vi "Apply Voltage.vi"(8 "error in (no error)":errorcluster, 10 "Number of Points":i32, 11 "Tool Path in":refnum<class "Tool Path.lvclass">) -> (0 "error out":errorcluster, 2 "Voltage Values":dbl[](array[numeric]), 3 "Tool Path out":refnum<class "Tool Path.lvclass">)   [LabVIEW 2019, in "Tool Path.lvclass"]
uses:
  Tool Path.lvclass
  subVIs/typedefs/Schedule - enum.ctl
  Settings/ObjectSettings/ObjectSettings.lvclass/ObjectSettings.ctl
  subVIs/typedefs/Schedule Types/Schedule--Constant.ctl
  subVIs/typedefs/Schedule Types/Schedule--Ramp.ctl
  subVIs/typedefs/Schedule Types/Schedule--Function Generator.ctl
  subVIs/typedefs/Schedule Types/Schedule--Formula.ctl
  Settings/Path Settings/Path Settings.lvclass
  C:/Users/Albro/Documents/GitHub/AFM-Lithography/lvsrc/Classes/Settings/ObjectSettings/ObjectSettings.lvclass
  <vilib>/Analysis/1siggen.llb/Ramp Pattern by Samples.vi
  Settings/ObjectSettings/ObjectSettings.lvclass
  <vilib>/Analysis/NI_AALBase.lvlib
  <vilib>/gmath/NI_Gmath.lvlib
  <vilib>/measure/NI_MABase.lvlib
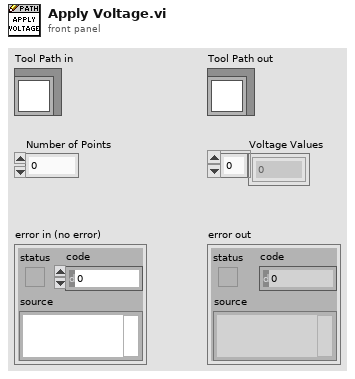
[diagram p1: front panel]
types:
  T1 = typedef "Schedule - enum.ctl" = enum16{"Constant", "Ramp", "Fn. Generator", "Formula"}
  T2 = enum16{"Sine Wave", "Triangle Wave", "Square Wave", "Sawtooth Wave"}
  T3 = typedef "Schedule--Constant.ctl" = cluster{"Value":dbl}
  T4 = typedef "Schedule--Ramp.ctl" = cluster{"Start":dbl, "End":dbl}
  T5 = typedef "Schedule--Function Generator.ctl" = cluster{"Min Value":dbl, "Max Value":dbl, "Duty Cycle (%)":dbl, "Signal Type":u16, "Cycle Number":dbl, "Phase (degrees)":dbl}
  T6 = typedef "Schedule--Formula.ctl" = cluster{"formula":string, "formula length (nm)":dbl, "formula resolution (nm)":dbl}
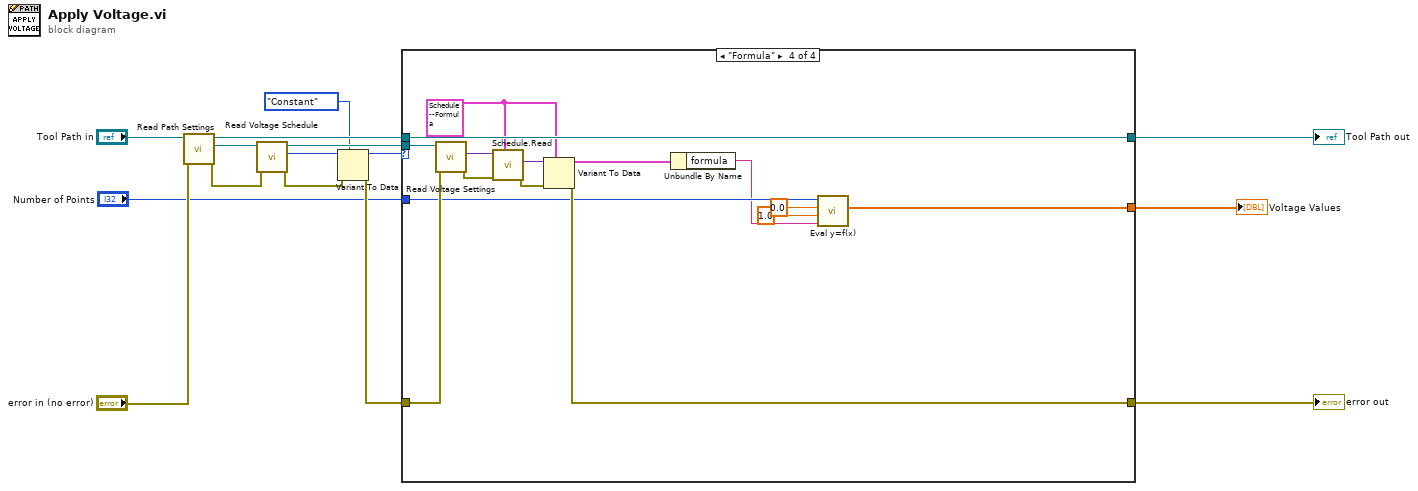
[diagram p0: block diagram]
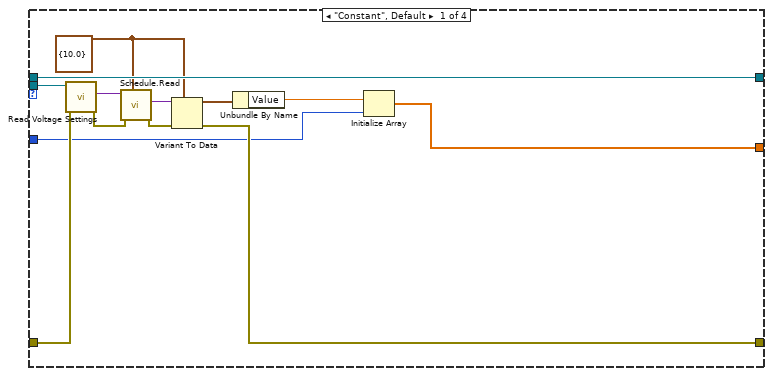
[diagram p2: hidden frame]
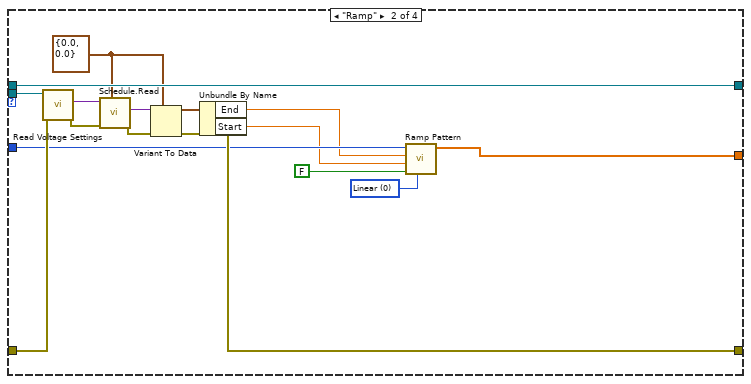
[diagram p3: hidden frame]
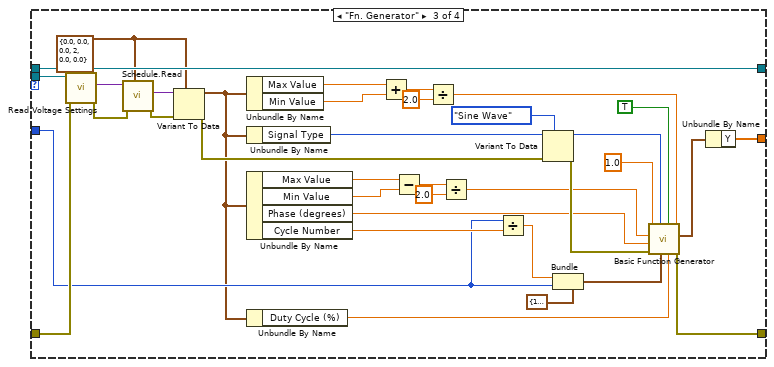
[diagram p4: hidden frame]
diagram:
  n1 = call-dynamic "Read Path Settings.vi"("error in (no error)"="error in (no error)", "Tool Path in"="Tool Path in") -> ("error out"=w4:errorcluster, "Path Settings.lvclass"=w13:refnum<class "Path Settings.lvclass">, "Tool Path out"=w11:refnum<class "Tool Path.lvclass">)  [unwired: 7 in]
  n2 = call "Read Voltage Schedule.vi"("error in (no error)"=w4, "ObjectSettings in"=w13) -> ("error out"=w3:errorcluster, "Schedule"=w7:u16, "ObjectSettings out"=w12:refnum<class "Path Settings.lvclass">)  [unwired: 7 in]
  n3 = Variant To Data(error in=w3, type=Schedule_-_enum."Constant" ("Schedule"), Variant=w7) -> (data=w6:T1, error out=w5:errorcluster)
  n4 = case shown="\"Formula\"" w6 {
    tunnel: w12 -> [w27 w44 w80 w95]
    tunnel: w11 -> [w28 w43 w79 w94]
    tunnel: [w28 w43 w79 w94] -> w10
    tunnel: w5 -> [w26 w42 w78 w93]
    tunnel: [w21 w38 w52 w86] -> w9
    tunnel: "Number of Points" -> [w17 w35 w53 w83]
    tunnel: [w16 w30 w46 w82] -> w1
    frame "Constant", Default {
      w20 = T3 {"Value"=10.0} ("Constant")
      n5 = call "Read Voltage Settings.vi"("error in (no error)"=w26, "ObjectSettings in"=w27) -> ("error out"=w24:errorcluster, "Settings"=w25:variant)  [unwired: 7 in, 1 out]
      n6 = call "Schedule.Read.vi"("Data to Read"=w20, "error in (no error)"=w24, "LUT In"=w25) -> ("error out"=w22:errorcluster, "Data Out"=w23:variant)  [unwired: 6 in, 1 out]
      n7 = Variant To Data(error in=w22, type=w20, Variant=w23) -> (data=w19:T3, error out=w21:errorcluster)
      n8 = Unbundle By Name(w19) -> ("Value"=w18:dbl)
      n9 = Initialize Array(w18, w17) -> (w16:dbl[])
    }
    frame "Ramp" {
      w34 = u16 0 items=["Linear", "Logarithmic"] ("type")
      w36 = T4 {"Start"=0.0, "End"=0.0} ("Ramp")
      n10 = call "Read Voltage Settings.vi"("error in (no error)"=w42, "ObjectSettings in"=w44) -> ("error out"=w39:errorcluster, "Settings"=w37:variant)  [unwired: 7 in, 1 out]
      n11 = call "Schedule.Read.vi"("Data to Read"=w36, "error in (no error)"=w39, "LUT In"=w37) -> ("error out"=w40:errorcluster, "Data Out"=w41:variant)  [unwired: 6 in, 1 out]
      n12 = Variant To Data(error in=w40, type=w36, Variant=w41) -> (data=w33:T4, error out=w38:errorcluster)
      n13 = Unbundle By Name(w33) -> ("End"=w29:dbl, "Start"=w32:dbl)
      n14 = call-poly <vilib>:"Ramp Pattern.vi"("type"=w34, "exclude end?"=FALSE, "start"=w32, "end"=w29, "samples"=w35) -> ("Ramp Pattern"=w30:dbl[])  [unwired: 5 in, 1 out]
    }
    frame "Fn. Generator" {
      w73 = T5 {"Min Value"=0.0, "Max Value"=0.0, "Duty Cycle (%)"=0.0, "Signal Type"=2, "Cycle Number"=0.0, "Phase (degrees)"=0.0} ("Fn. Gen")
      n15 = call "Read Voltage Settings.vi"("error in (no error)"=w78, "ObjectSettings in"=w80) -> ("error out"=w76:errorcluster, "Settings"=w75:variant)  [unwired: 7 in, 1 out]
      n16 = call "Schedule.Read.vi"("Data to Read"=w73, "error in (no error)"=w76, "LUT In"=w75) -> ("error out"=w77:errorcluster, "Data Out"=w74:variant)  [unwired: 6 in, 1 out]
      n17 = Variant To Data(error in=w77, type=w73, Variant=w74) -> (data=w47:T5, error out=w50:errorcluster)
      n18 = Unbundle By Name(w47) -> ("Max Value"=w54:dbl, "Min Value"=w55:dbl)
      n19 = Unbundle By Name(w47) -> ("Signal Type"=w64:u16)
      n20 = Unbundle By Name(w47) -> ("Max Value"=w60:dbl, "Min Value"=w61:dbl, "Phase (degrees)"=w49:dbl, "Cycle Number"=w68:dbl)
      n21 = Unbundle By Name(w47) -> ("Duty Cycle (%)"=w72:dbl)
      n22 = Add(x=w54, y=w55) -> (x+y=w56:dbl)
      n23 = Subtract(x=w60, y=w61) -> (x-y=w59:dbl)
      n24 = Divide(x=w56, y=2.0) -> (x/y=w62:dbl)
      n25 = Divide(x=w59, y=2.0) -> (x/y=w48:dbl)
      n26 = Divide(x=w53, y=w68) -> (x/y=w70:dbl)
      n27 = Variant To Data(error in=w50, type=T2."Sine Wave" ("signal type"), Variant=w64) -> (data=w66:T2, error out=w51:errorcluster)
      n28 = Bundle(cluster=cluster{"Fs":dbl, "#s":dbl} {"Fs"=1000.0, "#s"=1000.0} ("sampling info"), "Fs"=w70, "#s"=w53) -> (w71:cluster{"Fs":dbl, "#s":dbl})
      n29 = call <vilib>:"Basic Function Generator.vi"("offset"=w62, "square wave duty cycle (%)"=w72, "reset signal"=TRUE, "sampling info"=w71, "signal type"=w66, "error in (no error)"=w51, "phase"=w49, "amplitude"=w48, "frequency"=1.0) -> ("error out"=w52:errorcluster, "signal out"=w45:waveform(dbl))  [unwired: 1 out]
      n30 = Unbundle By Name(w45) -> ("Y"=w46:dbl[])
    }
    frame "Formula" {
      w89 = T6 {"formula"="1*(step(170-t)*cos(0.62831853071*t)+step(t-170)*cos(0.62831853071*(t-170))*(-1))", "formula length (nm)"=340.0, "formula resolution (nm)"=0.001} ("Formula")
      n31 = call "Read Voltage Settings.vi"("error in (no error)"=w93, "ObjectSettings in"=w95) -> ("error out"=w90:errorcluster, "Settings"=w91:variant)  [unwired: 7 in, 1 out]
      n32 = call "Schedule.Read.vi"("Data to Read"=w89, "error in (no error)"=w90, "LUT In"=w91) -> ("error out"=w92:errorcluster, "Data Out"=w88:variant)  [unwired: 6 in, 1 out]
      n33 = Variant To Data(error in=w92, type=w89, Variant=w88) -> (data=w87:T6, error out=w86:errorcluster)
      n34 = Unbundle By Name(w87) -> ("formula"=w81:string)
      n35 = call <vilib>:"Eval y=f(x).vi"("formula"=w81, "end"=1.0, "start"=0.0, "number of points"=w83) -> ("Y Values"=w82:dbl[])  [unwired: 3 out]
    }
  }
  "error out" <- w9
  "Tool Path out" <- w10
  "Voltage Values" <- w1
